vi "Error Query.vi"(8 "error in (no error)":errorcluster, 11 "VISA resource name":refnum<visa-resource-name>) -> (0 "error out":errorcluster, 1 "Error Message":string, 3 "VISA resource name out":refnum<visa-resource-name>)   [LabVIEW 2021, in "BK Precision 5491B.lvlib"]
doc: "Queries the instrument for any errors in the instrument's error queue. It will continue to read errors until all errors have been read from the instrument. Any errors will be returned in the <B>error out</B> control.\n\n<B>Note:</B>\nThis VI is called automatically by most driver VIs so it is not usually necessary to call this in an application."
uses:
  <instrlib>/BK Precision 5491B/BK Precision 5491B.lvlib
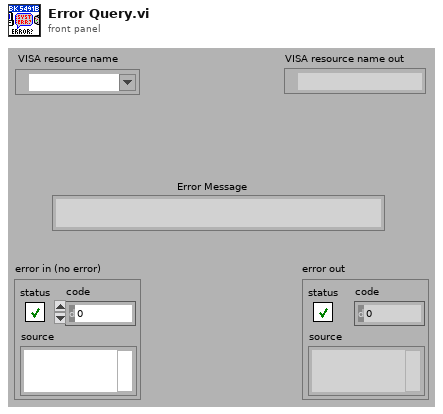
[diagram p1: front panel]
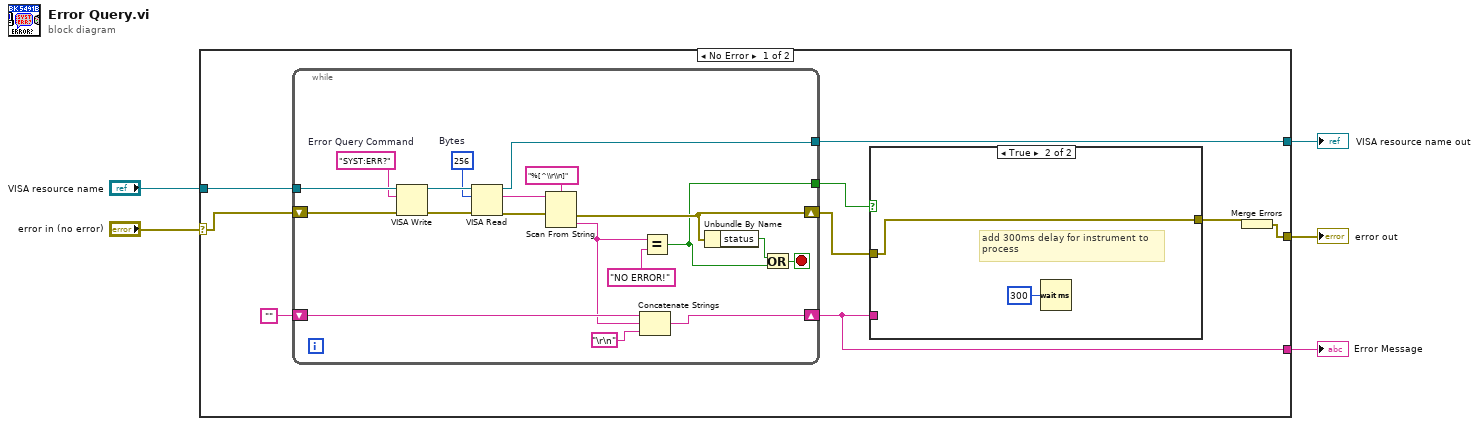
[diagram p0: block diagram]
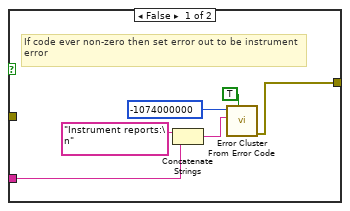
[diagram p2: hidden frame]
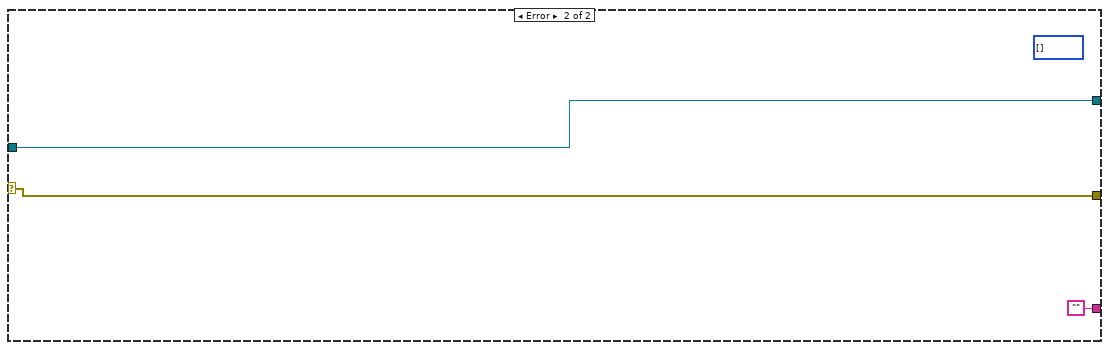
[diagram p3: hidden frame]
diagram:
  n1 = case shown="No Error" "error in (no error)" {
    selector: "error in (no error)" -> [w7 w42]
    tunnel: [w14 w44] -> w5
    tunnel: "VISA resource name" -> [w13 w44]
    tunnel: [w11 w42] -> w4
    tunnel: [w9 ""] -> w3
    frame No Error {
      n2 = while {
        tunnel: [w41] -> w14
        tunnel: w13 -> [w40]
        shift-right: [w30] -> w9
        shift-left: "" -> [w32]
        shift-right: [w26] -> w8
        shift-left: w7 -> [w29]
        tunnel: [w23] -> w6
        stop <- w35 stop-if-true
        w38 = u32 256  # Bytes
        w36 = "SYST:ERR?"  # Error Query Command
        n3 = VISA Write(VISA resource name=w40, write buffer=w36, error in (no error)=w29) -> (VISA resource name out=w39:refnum<visa-resource-name>, error out=w37:errorcluster)  [unwired: 1 out]
        n4 = VISA Read(VISA resource name=w39, byte count=w38, error in (no error)=w37) -> (VISA resource name out=w41:refnum<visa-resource-name>, read buffer=w33:string, error out=w28:errorcluster)  [unwired: 1 out]
        n5 = Scan From String(format string="%[^\\r\\n]", input string=w33, error in=w28) -> (error out=w26:errorcluster, output 1=w25:string)  [unwired: 2 in, 2 out]
        n6 = Concatenate Strings(w32, w25, "\r\n") -> (w30:string)
        n7 = Equal?(x=w25, y="NO ERROR!") -> (x = y?=w23:bool)
        n8 = Unbundle By Name(w26) -> ("status"=w27:bool)
        n9 = Or(x=w27, y=w23) -> (x .or. y?=w35:bool)
      }
      n10 = case shown="True" w6 {
        tunnel: w9 -> [w19 _]
        tunnel: [w15 w22] -> w10
        tunnel: w8 -> [_ w22]
        frame False {
          # "If code ever non-zero then set error out to be instrument error"
          n11 = Concatenate Strings("Instrument reports:\n" ("Source"), w19) -> (w16:string)
          n12 = call <vilib>:"Error Cluster From Error Code.vi"("show call chain? (False)"=TRUE, "error message (\"\")"=w16, "error code (0)"=-1074000000 ("Code")) -> ("error out"=w15:errorcluster)  [unwired: 6 in]
        }
        frame True {
          # "add 300ms delay for instrument to\nprocess"
          n13 = Wait (ms)(milliseconds to wait=u32 300) -> ()  [unwired: 1 out]
        }
      }
      n14 = Merge Errors(w10) -> (w11:errorcluster)
    }
    frame Error {
      (unwired) i32[] []
    }
  }
  "VISA resource name out" <- w5
  "error out" <- w4
  "Error Message" <- w3
